vi "cs_isStimListValid.vi"(8 "error in (no error)":errorcluster, 11 "Array":dbl[][](array[numeric])) -> (0 "error out":errorcluster, 3 "Valid?":bool)   [LabVIEW 2013]
uses:
  <vilib>/Utility/error.llb/DialogType.ctl
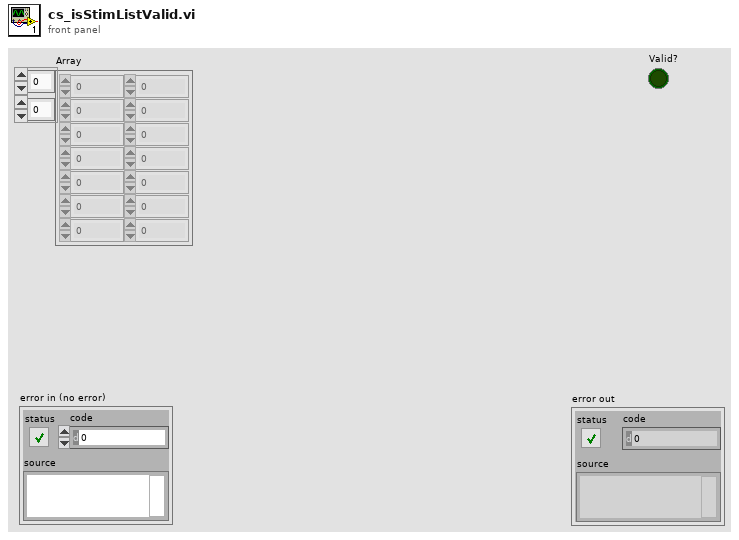
[diagram p1: front panel]
types:
  T1 = typedef "DialogType.ctl" = u16
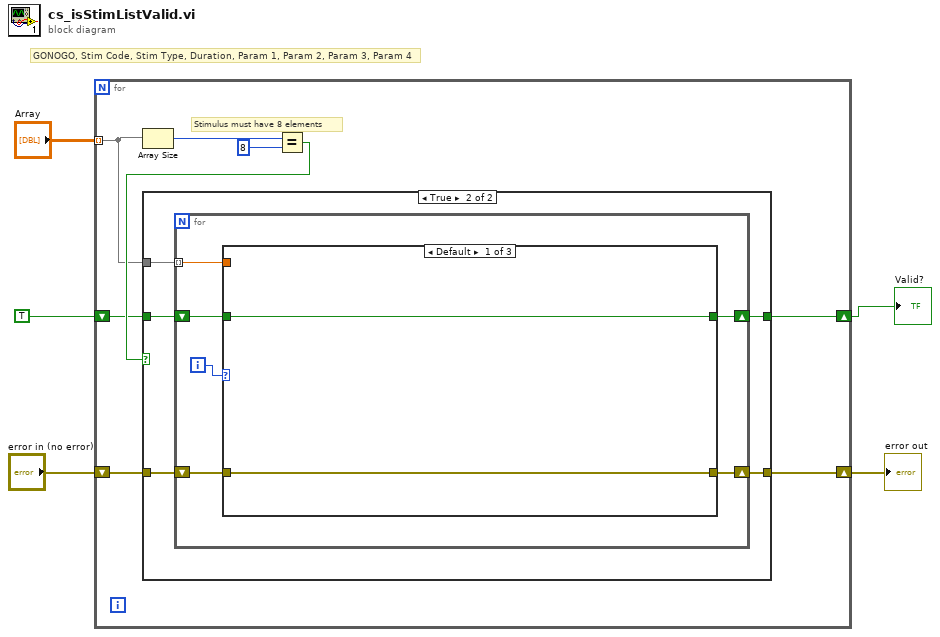
[diagram p0: block diagram]
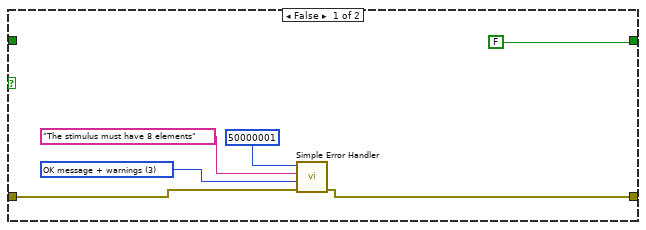
[diagram p2: hidden frame]
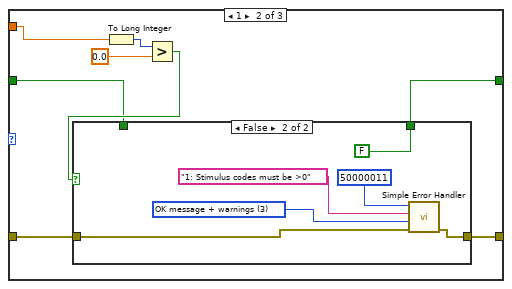
[diagram p3: hidden frame]
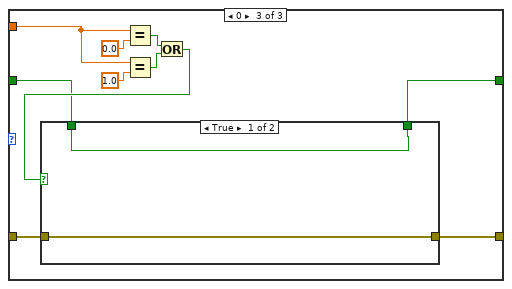
[diagram p5: hidden frame]
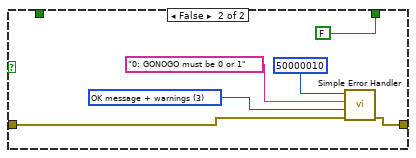
[diagram p6: hidden frame]
diagram:
  # "GONOGO, Stim Code, Stim Type, Duration, Param 1, Param 2, Param 3, Param 4"
  n1 = for {
    tunnel: "Array" -> [w10] mode=indexing
    shift-right: [w8] -> w3
    shift-left: "error in (no error)" -> [w9]
    shift-right: [w6] -> w1
    shift-left: TRUE -> [w7]
    # "Stimulus must have 8 elements"
    n2 = Array Size(array=w10) -> (size(s)=w12:i32)
    n3 = Equal?(x=w12, y=8) -> (x = y?=w11:bool)
    n4 = case shown="True" w11 {
      tunnel: w10 -> [_ w22]
      tunnel: w9 -> [w19 w24]
      tunnel: [w16 w23] -> w8
      tunnel: w7 -> [_ w21]
      tunnel: [FALSE w20] -> w6
      frame False {
        w18 = T1 3 items=["no dialog", "OK message", "continue or stop message", "OK message + warnings", "continue/stop + warnings"] ("type of dialog (OK msg:1)")
        n5 = call <vilib>:"Simple Error Handler.vi"("error code (no error:0)"=50000001, "error source (\" \")"="The stimulus must have 8 elements" ("error source (\" \")"), "type of dialog (OK msg:1)"=w18, "error in (no error)"=w19) -> ("error out"=w16:errorcluster)  [unwired: 1 in, 4 out]
      }
      frame True {
        n6 = for {
          shift-right: [w28] -> w23
          shift-left: w24 -> [w29]
          tunnel: w22 -> [w30] mode=indexing
          shift-right: [w25] -> w20
          shift-left: w21 -> [w26]
          i -> [w27]
          n7 = case shown="Default" w27 {
            tunnel: w30 -> [_ w38 w54]
            tunnel: w29 -> [w32 w36 w53]
            tunnel: [w32 w33 w52] -> w28
            tunnel: w26 -> [w31 w35 w50]
            tunnel: [w31 w34 w49] -> w25
            frame Default {
            }
            frame 1 {
              n8 = To Long Integer(number=w38) -> (32bit integer=w40:i32)
              n9 = Greater?(x=w40, y=0.0) -> (0:w37:bool)
              n10 = case shown="False" w37 {
                tunnel: w36 -> [w42 w45]
                tunnel: [w42 w44] -> w33
                tunnel: w35 -> [w41 _]
                tunnel: [w41 FALSE] -> w34
                frame True {
                }
                frame False {
                  w48 = T1 3 items=["no dialog", "OK message", "continue or stop message", "OK message + warnings", "continue/stop + warnings"] ("type of dialog (OK msg:1)")
                  n11 = call <vilib>:"Simple Error Handler.vi"("error code (no error:0)"=50000011, "error source (\" \")"="1: Stimulus codes must be >0" ("error source (\" \")"), "type of dialog (OK msg:1)"=w48, "error in (no error)"=w45) -> ("error out"=w44:errorcluster)  [unwired: 1 in, 4 out]
                }
              }
            }
            frame 0 {
              n12 = Equal?(x=w54, y=0.0) -> (x = y?=w57:bool)
              n13 = Equal?(x=w54, y=1.0) -> (x = y?=w58:bool)
              n14 = Or(x=w57, y=w58) -> (x .or. y?=w51:bool)
              n15 = case shown="True" w51 {
                tunnel: w53 -> [w60 w63]
                tunnel: [w60 w62] -> w52
                tunnel: w50 -> [w59 _]
                tunnel: [w59 FALSE] -> w49
                frame True {
                }
                frame False {
                  w66 = T1 3 items=["no dialog", "OK message", "continue or stop message", "OK message + warnings", "continue/stop + warnings"] ("type of dialog (OK msg:1)")
                  n16 = call <vilib>:"Simple Error Handler.vi"("error code (no error:0)"=50000010, "error source (\" \")"="0: GONOGO must be 0 or 1" ("error source (\" \")"), "type of dialog (OK msg:1)"=w66, "error in (no error)"=w63) -> ("error out"=w62:errorcluster)  [unwired: 1 in, 4 out]
                }
              }
            }
          }
        }
      }
    }
  }
  "Valid?" <- w1
  "error out" <- w3
